vi "MANEJO TURNOS.vi"() -> ()   [LabVIEW 2020, in "Manejador Turnos.lvlib"]
uses:
  Manejador Turnos.lvlib
panel:
  in  "Lista servicios":string[][](array[string])
  in  "Multicolumn Listbox":i32(listbox)
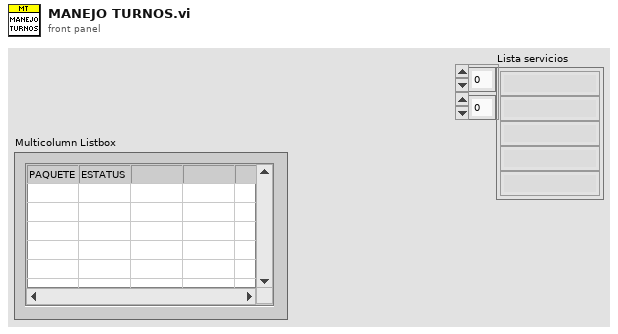
[diagram p1: front panel]
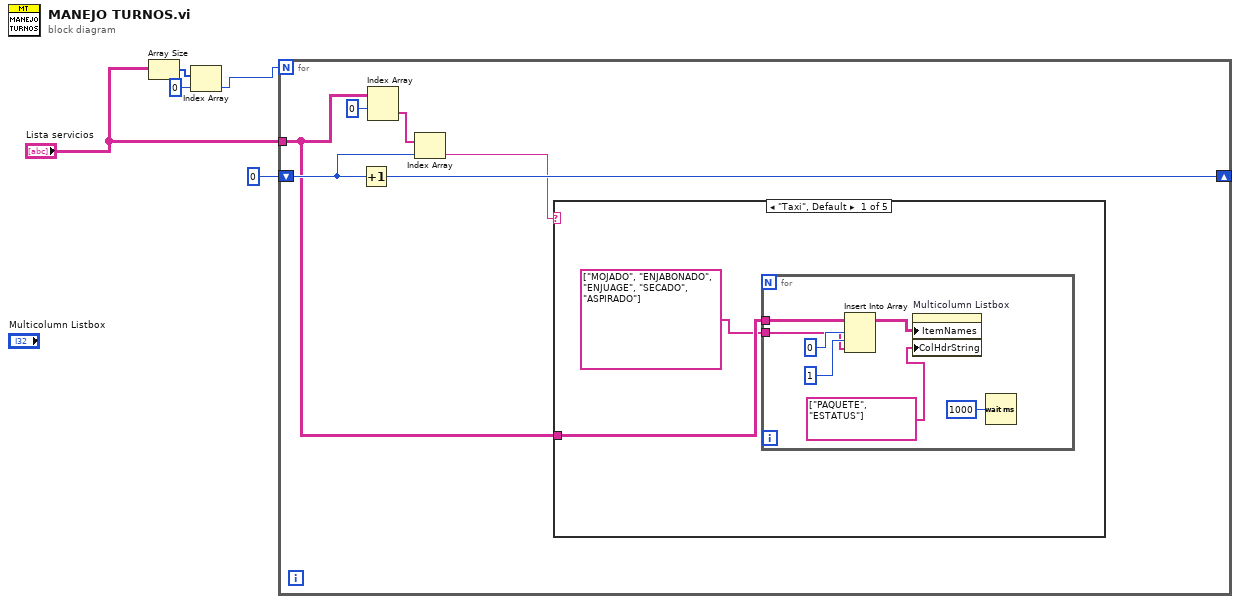
[diagram p0: block diagram]
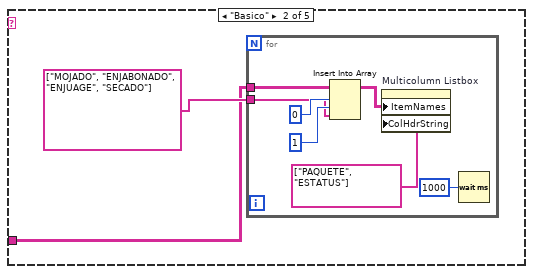
[diagram p2: hidden frame]
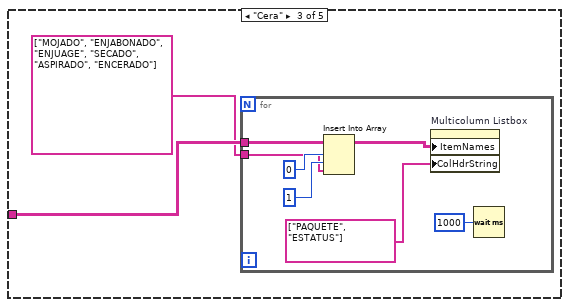
[diagram p3: hidden frame]
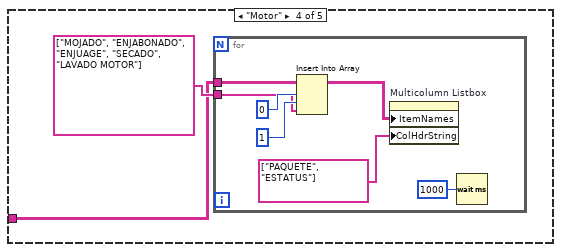
[diagram p4: hidden frame]
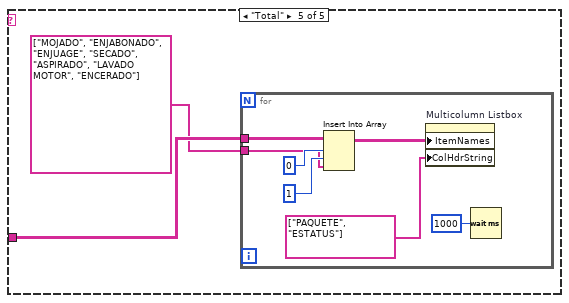
[diagram p5: hidden frame]
diagram:
  n1 = Array Size(array="Lista servicios") -> (size(s)=w3:i32[])
  n2 = Index Array(array=w3, index=0) -> (element=w1:i32)
  n3 = for {
    N: w1 -> [_]
    tunnel: "Lista servicios" -> [w6]
    shift-right: [w10] -> _
    shift-left: 0 ("index") -> [w11]
    n4 = Increment(x=w11) -> (x+1=w10:i32)
    n5 = Index Array(array=w6, index (row)=0) -> (element=w7:string[])  [unwired: 1 in]
    n6 = Index Array(array=w7, index=w11) -> (element=w9:string)
    n7 = case shown="\"Taxi\", Default" w9 {
      tunnel: w6 -> [w13 w21 w31 w39 w49]
      frame "Taxi", Default {
        n8 = for {
          tunnel: w13 -> [w20]
          tunnel: string[] ["MOJADO", "ENJABONADO", "ENJUAGE", "SECADO", "ASPIRADO"] -> [w17]
          n9 = Insert Into Array(array=w20, index (row)=0, index (col)=1 ("disabled index (col)"), new element=w17) -> (w16:string[][])
          n10 = property on="Multicolumn Listbox" class="MCListbox (strict)"("ItemNames"=w16, "ColHdrString"=string[] ["PAQUETE", "ESTATUS"] ("Column Header Strings[]")) -> ()  [unwired: 2 in, 2 out]
          n11 = Wait (ms)(milliseconds to wait=u32 1000) -> ()  [unwired: 1 out]
        }
      }
      frame "Basico" {
        n12 = for {
          tunnel: w21 -> [w29]
          tunnel: string[] ["MOJADO", "ENJABONADO", "ENJUAGE", "SECADO"] -> [w26]
          n13 = Insert Into Array(array=w29, index (row)=0, index (col)=1 ("disabled index (col)"), new element=w26) -> (w25:string[][])
          n14 = property on="Multicolumn Listbox" class="MCListbox (strict)"("ItemNames"=w25, "ColHdrString"=string[] ["PAQUETE", "ESTATUS"] ("Column Header Strings[]")) -> ()  [unwired: 2 in, 2 out]
          n15 = Wait (ms)(milliseconds to wait=u32 1000) -> ()  [unwired: 1 out]
        }
      }
      frame "Cera" {
        n16 = for {
          tunnel: w31 -> [w38]
          tunnel: string[] ["MOJADO", "ENJABONADO", "ENJUAGE", "SECADO", "ASPIRADO", "ENCERADO"] -> [w35]
          n17 = Insert Into Array(array=w38, index (row)=0, index (col)=1 ("disabled index (col)"), new element=w35) -> (w33:string[][])
          n18 = property on="Multicolumn Listbox" class="MCListbox (strict)"("ItemNames"=w33, "ColHdrString"=string[] ["PAQUETE", "ESTATUS"] ("Column Header Strings[]")) -> ()  [unwired: 2 in, 2 out]
          n19 = Wait (ms)(milliseconds to wait=u32 1000) -> ()  [unwired: 1 out]
        }
      }
      frame "Motor" {
        n20 = for {
          tunnel: w39 -> [w47]
          tunnel: string[] ["MOJADO", "ENJABONADO", "ENJUAGE", "SECADO", "LAVADO MOTOR"] -> [w44]
          n21 = Insert Into Array(array=w47, index (row)=0, index (col)=1 ("disabled index (col)"), new element=w44) -> (w42:string[][])
          n22 = property on="Multicolumn Listbox" class="MCListbox (strict)"("ItemNames"=w42, "ColHdrString"=string[] ["PAQUETE", "ESTATUS"] ("Column Header Strings[]")) -> ()  [unwired: 2 in, 2 out]
          n23 = Wait (ms)(milliseconds to wait=u32 1000) -> ()  [unwired: 1 out]
        }
      }
      frame "Total" {
        n24 = for {
          tunnel: w49 -> [w56]
          tunnel: string[] ["MOJADO", "ENJABONADO", "ENJUAGE", "SECADO", "ASPIRADO", "LAVADO MOTOR", "ENCERADO"] -> [w53]
          n25 = Insert Into Array(array=w56, index (row)=0, index (col)=1 ("disabled index (col)"), new element=w53) -> (w51:string[][])
          n26 = property on="Multicolumn Listbox" class="MCListbox (strict)"("ItemNames"=w51, "ColHdrString"=string[] ["PAQUETE", "ESTATUS"] ("Column Header Strings[]")) -> ()  [unwired: 2 in, 2 out]
          n27 = Wait (ms)(milliseconds to wait=u32 1000) -> ()  [unwired: 1 out]
        }
      }
    }
  }
